vi "Simulator Start.vi"() -> ()   [LabVIEW 2017, in "XYStage.KIM101.lvclass"]
uses:
  XYStage.KIM101.lvclass
  D:/upwork/Laser Measurement Tool/Laser/project/data/Thorlabs.MotionControl.DeviceManagerCLI.dll
  data/Thorlabs.MotionControl.DeviceManagerCLI.dll
panel:
  out "error out":errorcluster
  in  "Serial Number":string="97000001"
  # "START"
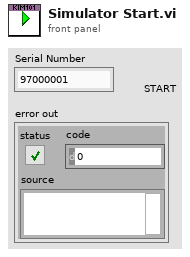
[diagram p1: front panel]
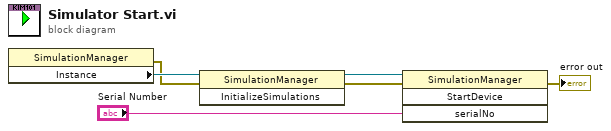
[diagram p0: block diagram]
diagram:
  n1 = property class="SimulationManager"() -> (error out=w4:errorcluster, "Instance"=w6:refnum<k24>)  [unwired: 2 in, 1 out]
  n2 = invoke class="SimulationManager" method="InitializeSimulations"(reference=w6, error in=w4) -> (reference out=w5:refnum<k24>, error out=w3:errorcluster)  [unwired: 1 in, 1 out]
  n3 = invoke class="SimulationManager" method="StartDevice"(reference=w5, error in=w3, "serialNo"="Serial Number") -> (error out=→"error out":errorcluster)  [unwired: 1 in, 3 out]
